vi "Cal Curent Week.vi"() -> (0 "CurWeek(0)":i32)   [LabVIEW 2015, in "CalAttendance.lvclass"]
uses:
  CalAttendance.lvclass
  Setting/g_setting.vi
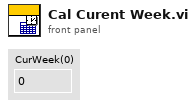
[diagram p1: front panel]
types:
  T1 = typedef "LVDateTimeRec.ctl" = cluster{"fractional second":dbl, "second":i32, "minute":i32, "hour":i32, "day of month":i32, "month":i32, "year":i32, "day of week":i32, "day of year":i32, "DST":i32}
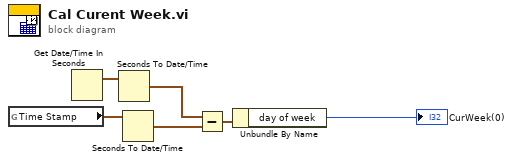
[diagram p0: block diagram]
diagram:
  n1 = global read "g_setting.vi" "Time Stamp"() -> (w4:timestamp)
  n2 = Get Date/Time In Seconds() -> (seconds since 1Jan1904=w2:timestamp)
  n3 = Seconds To Date/Time(time stamp (now)=w2) -> (date time rec=w3:T1)  [unwired: 1 in]
  n4 = Seconds To Date/Time(time stamp (now)=w4) -> (date time rec=w5:T1)  [unwired: 1 in]
  n5 = Subtract(x=w3, y=w5) -> (x-y=w6:T1)
  n6 = Unbundle By Name(w6) -> ("day of week"=→"CurWeek(0)":i32)
